vi "Read States.vi"(8 "error in (no error)":errorcluster, 11 "5RobotsTactic in":refnum<class "5RobotsTactic.lvclass">) -> (0 "error out":errorcluster, 2 "States":enum16{"Position", "Exit"}(ring), 3 "5RobotsTactic out":refnum<class "5RobotsTactic.lvclass">)   [LabVIEW 2020, in "5RobotsTactic.lvclass"]
uses:
  5RobotsTactic.lvclass
  5RobotsTactic.lvclass/5RobotsTactic.ctl
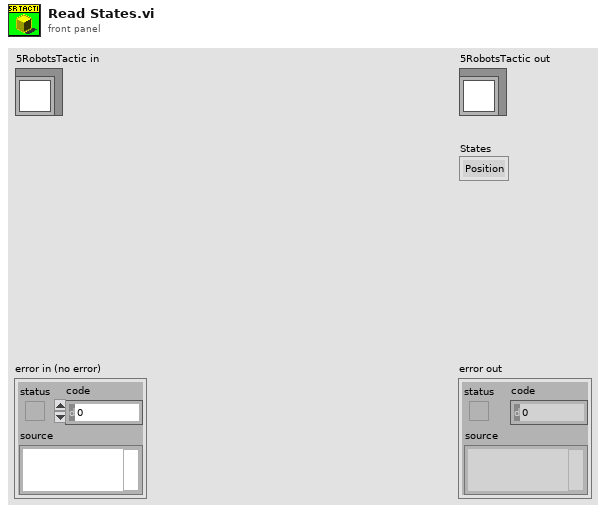
[diagram p1: front panel]
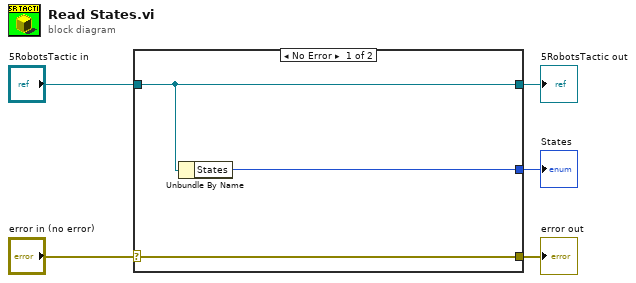
[diagram p0: block diagram]
diagram:
  n1 = case shown="No Error" "error in (no error)" {
    selector: "error in (no error)" -> [w8 w9]
    tunnel: [w8 w9] -> w4
    tunnel: [w7 w10] -> w2
    tunnel: "5RobotsTactic in" -> [w7 w10]
    tunnel: [w6 _] -> w1
    frame No Error {
      n2 = Unbundle By Name(w7) -> ("States"=w6:enum16{"Position", "Exit"})
    }
    frame Error {
    }
  }
  "error out" <- w4
  "5RobotsTactic out" <- w2
  "States" <- w1
